vi "Cleanup.vi"(8 "error in (no error)":errorcluster, 11 "Agent_Inv In":refnum<class "Agent.lvclass">) -> (0 "error out":errorcluster)   [LabVIEW 2019, in "Agent.lvclass"]
doc: "Clean up after Agent. Closes the order queue"
uses:
  Agent.lvclass
  Agent.lvclass/Agent.ctl
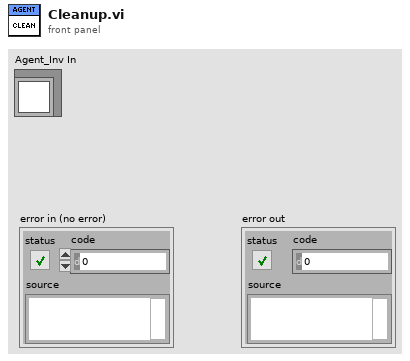
[diagram p1: front panel]
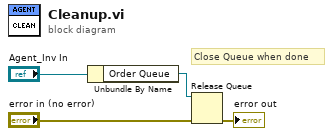
[diagram p0: block diagram]
diagram:
  # "Close Queue when done"
  n1 = Unbundle By Name("Agent_Inv In") -> ("Order Queue"=w3:refnum<queue>)
  n2 = Release Queue(queue=w3, error in (no error)="error in (no error)") -> (error out=→"error out":errorcluster)  [unwired: 1 in, 2 out]
